vi "Read stream.vi"(8 "error in (no error)":errorcluster, 11 "TextTestRunner in":refnum<class "TextTestRunner.lvclass">) -> (0 "error out":errorcluster, 2 "stream":refnum<queue>, 3 "TextTestRunner out":refnum<class "TextTestRunner.lvclass">)   [LabVIEW 2013, in "TextTestRunner.lvclass"]
uses:
  TextTestRunner.lvclass
  TextTestRunner.lvclass/TextTestRunner.ctl
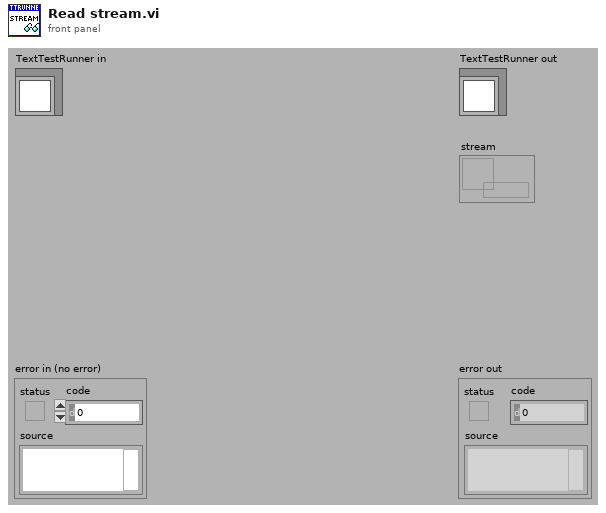
[diagram p1: front panel]
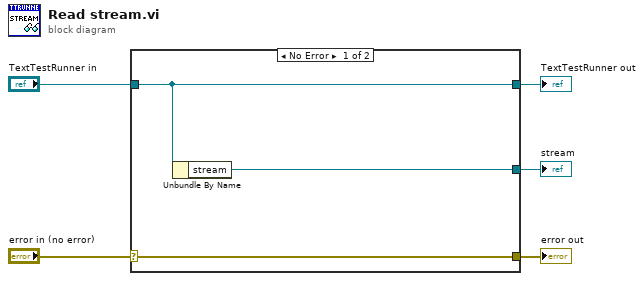
[diagram p0: block diagram]
diagram:
  n1 = case shown="No Error" "error in (no error)" {
    selector: "error in (no error)" -> [w8 w9]
    tunnel: [w8 w9] -> w4
    tunnel: [w7 w10] -> w2
    tunnel: "TextTestRunner in" -> [w7 w10]
    tunnel: [w6 _] -> w1
    frame No Error {
      n2 = Unbundle By Name(w7) -> ("stream"=w6:refnum<queue>)
    }
    frame Error {
    }
  }
  "error out" <- w4
  "TextTestRunner out" <- w2
  "stream" <- w1
